vi "配置文件路径.vi"(8 "error in (no error)":errorcluster, 11 "TimingControl 输入":refnum<class "TimingControl.lvclass">) -> (0 "error out":errorcluster, 3 "TimingControl 输出":refnum<class "TimingControl.lvclass">)   [LabVIEW 2016, in "TimingControl.lvlib" / "TimingControl.lvclass"]
uses:
  TimingControl.lvclass
  TimingControl.lvclass/TimingControl.ctl
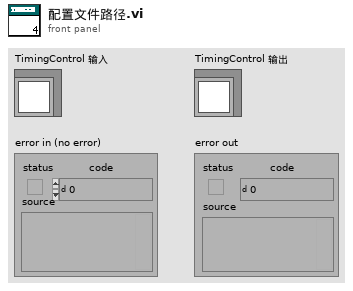
[diagram p1: front panel]
types:
  T1 = typedef "TimingControl.lvlib/TimingControl.lvclass/State Data.ctl" = cluster{"仪器时间":timestamp, "仪器运行状态":bool, "配置文件路径":path, "测量参数":u16, "测试状态":cluster{"启动时间":timestamp, "结束时间":timestamp, "启动次数":dbl}, "配置信息":T2}
  T2 = typedef "TimingControl.lvlib/TimingControl.lvclass/配置信息.ctl" = cluster{"每周启动":T3, "每月启动":T4, "周期模式":T5, "测量参数":T6, "定点周期":T7, "间隔启动":T9, "配置时间":timestamp}
  T3 = typedef "TimingControl.lvlib/TimingControl.lvclass/每周启动.ctl" = enum16{"关闭", "周日", "周一", "周二", "周三", "周四", "周五", "周六"}
  T4 = typedef "TimingControl.lvlib/TimingControl.lvclass/每月启动.ctl" = enum16{"关闭", "1号", "2号", "3号", "4号", "5号", "6号", "7号", "8号", "9号", "10号", "11号", "12号", "13号", "14号", "15号", "16号", "17号", "18号", "19号", "20号", "21号", "22号", "23号", "24号", "25号", "26号", "27号", "28号", "29号", "30号", "31号"}
  T5 = typedef "TimingControl.lvlib/TimingControl.lvclass/周期模式设置.ctl" = enum16{"不启用", "定点模式", "间隔模式"}
  T6 = typedef "TimingControl.lvlib/TimingControl.lvclass/测量参数.ctl" = u16
  T7 = typedef "TimingControl.lvlib/TimingControl.lvclass/定点周期设置.ctl" = cluster{"启动命令":T8, "启动命令 2":T8, "启动命令 3":T8, "启动命令 4":T8, "启动命令 5":T8, "启动命令 6":T8, "启动命令 7":T8, "启动命令 8":T8, "启动命令 9":T8, "启动命令 10":T8, "启动命令 11":T8, "启动命令 12":T8, "启动命令 13":T8, "启动命令 14":T8, "启动命令 15":T8, "启动命令 16":T8, "启动命令 17":T8, "启动命令 18":T8, "启动命令 19":T8, "启动命令 20":T8, "启动命令 21":T8, "启动命令 22":T8, "启动命令 23":T8, "启动命令 24":T8}
  T8 = typedef "TimingControl.lvlib/TimingControl.lvclass/启动命令选择.ctl" = enum16{"", "水样测试", "标样核查", "零点核查", "跨度核查", "空白测试", "平行样测试", "加标回收", "空白校准", "标样校准", "初始化(清洗)"}
  T9 = typedef "TimingControl.lvlib/TimingControl.lvclass/间隔启动设置.ctl" = cluster{"启动命令":T8, "启动间隔":dbl, "启动次数":i32}
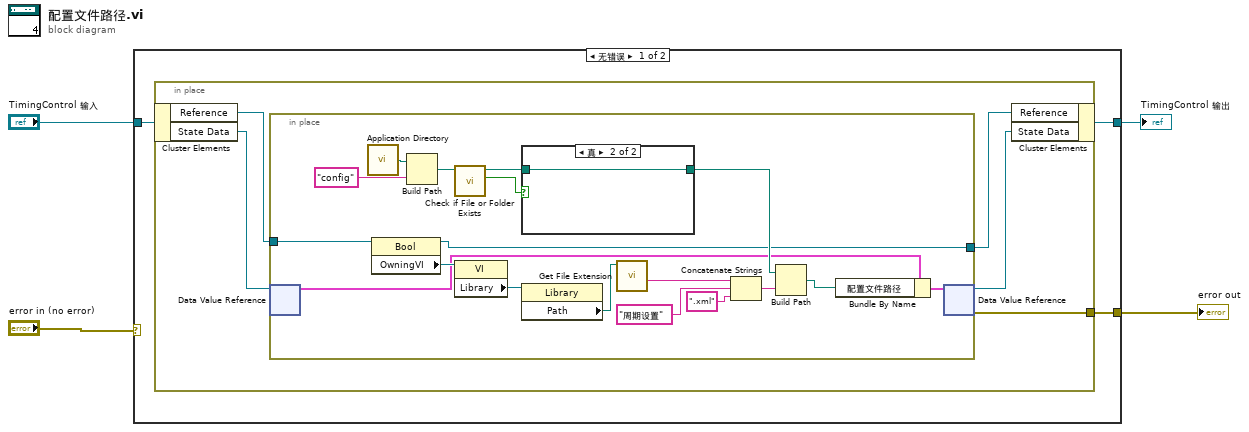
[diagram p0: block diagram]
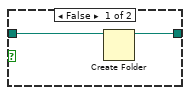
[diagram p2: hidden frame]
diagram:
  n1 = case shown="无错误" "error in (no error)" {
    selector: "error in (no error)" -> [_ w35]
    tunnel: "TimingControl 输入" -> [w7 w34]
    tunnel: [w6 w34] -> w3
    tunnel: [w5 w35] -> w1
    frame No Error {
      n2 = in-place {
        in-place-border: [w8] -> w5
        n3 = in-place-cluster #1(w7) -> ("Reference"=w12:refnum<vi>, "State Data"=w10:refnum<data-value>)
        n4 = in-place {
          in-place-border: w12 -> [w19]
          in-place-border: [w18] -> w11
          n5 = in-place-dvr #2(w10) -> (w17:T1)  [unwired: 1 out]
          n6 = call <vilib>:"Application Directory.vi"() -> ("Application Directory"=w27:path)
          n7 = property class="Bool"(reference=w19) -> (reference out=w18:refnum<vi>, "OwningVI"=w29:refnum<vi>)  [unwired: 1 in, 1 out]
          n8 = Build Path(base path=w27, name or relative path="config" ("名称或相对路径")) -> (appended path=w25:path)
          n9 = call <vilib>:"Check if File or Folder Exists.vi"("path"=w25) -> ("file or folder exists?"=w22:bool, "dup path"=w21:path)  [unwired: 8 in, 1 out]
          n10 = property class="VI"(reference=w29) -> ("Library"=w30:refnum<vi>)  [unwired: 1 in, 2 out]
          n11 = case shown="真" w22 {
            tunnel: w21 -> [w32 w33]
            tunnel: [w31 w33] -> w20
            frame False {
              n12 = Create Folder(path (use dialog)=w32) -> (created path=w31:path)  [unwired: 2 in, 2 out]
            }
            frame True {
            }
          }
          n13 = property class="Library"(reference=w30) -> ("Path"=w28:path)  [unwired: 1 in, 2 out]
          n14 = call <vilib>:"Get File Extension.vi"("file"=w28) -> ("filename without extension"=w14:string)  [unwired: 6 in, 4 out]
          n15 = Concatenate Strings(w14, "周期设置" ("字符串"), ".xml" ("字符串")) -> (w23:string)
          n16 = Build Path(base path=w20, name or relative path=w23) -> (appended path=w15:path)
          n17 = Bundle By Name(cluster=w17, "配置文件路径"=w15) -> (w16:T1)
          n18 = in-place-dvr #2(w16) -> (w9:refnum<data-value>, w8:errorcluster)
        }
        n19 = in-place-cluster #1("Reference"=w11, "State Data"=w9) -> (w6:refnum<class "TimingControl.lvclass">)
      }
    }
    frame Error {
    }
  }
  "TimingControl 输出" <- w3
  "error out" <- w1
